vi "Status Log FGV.vi"(7 "Action":T1=enum."Show Status File", 8 "error in":errorcluster, 10 "Status":string) -> (0 "error out":errorcluster)   [LabVIEW 2016]
doc: "FGV for managing status log file"
uses:
  Status Log.ctl
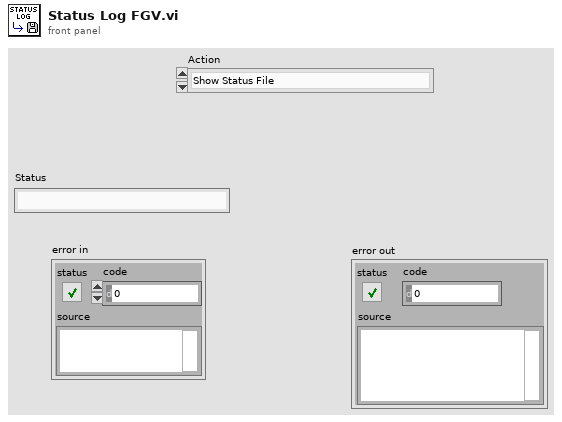
[diagram p1: front panel]
types:
  T1 = typedef "Status Log.ctl" = enum16{"Close file", "Open Status file", "Add Status", "Show Status File"}
  T2 = enum16{"open", "replace", "create", "open or create", "replace or create", "replace or create with confirmation"}
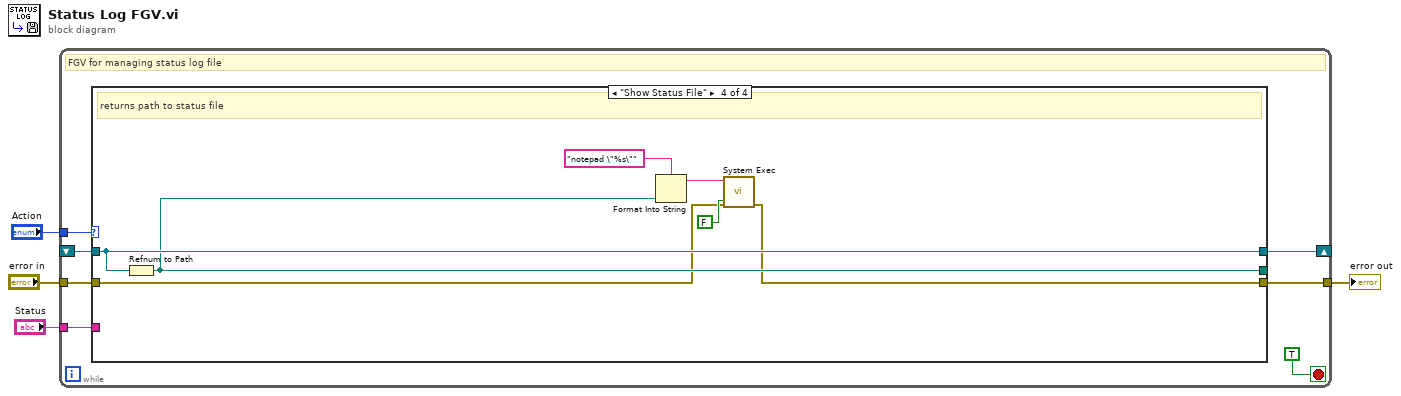
[diagram p0: block diagram]
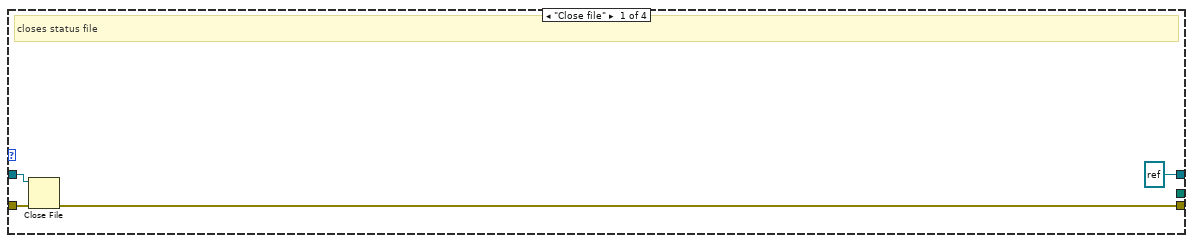
[diagram p2: hidden frame]
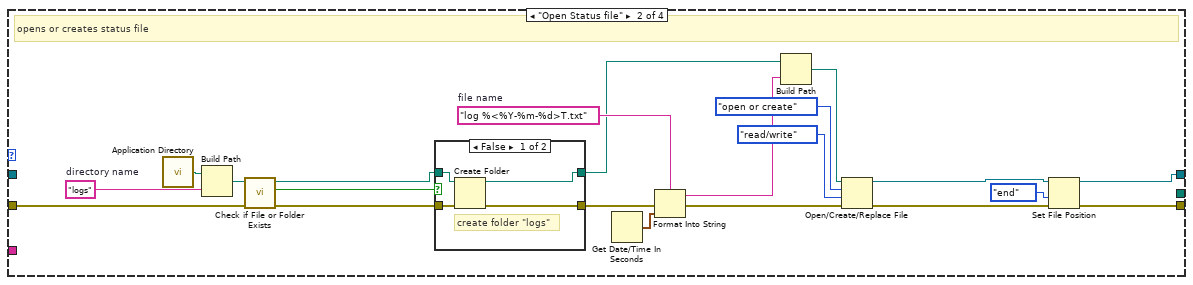
[diagram p3: hidden frame]
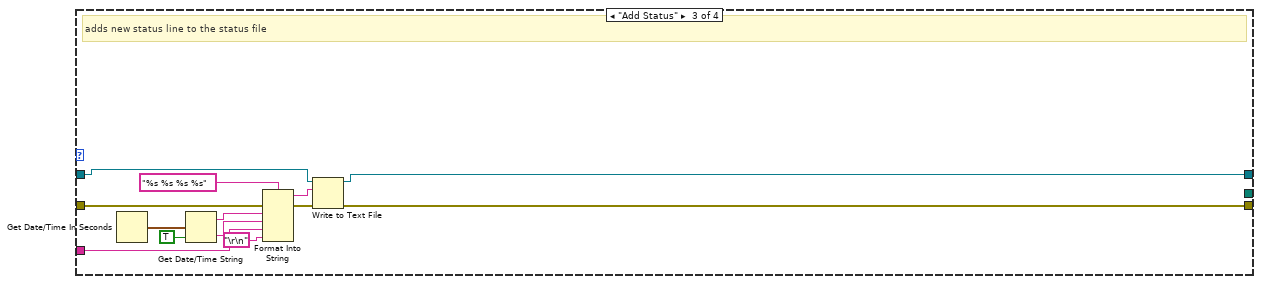
[diagram p5: hidden frame]
diagram:
  n1 = while {
    tunnel: "Action" -> [w10]
    tunnel: "Status" -> [w9]
    tunnel: [w8] -> w2
    tunnel: "error in" -> [w7]
    shift-right: [w5] -> _
    shift-left: _ -> [w6]
    stop <- TRUE stop-if-true
    # "FGV for managing status log file"
    n2 = case shown="\"Show Status File\"" w10 {
      tunnel: w9 -> [_ _ w49 _]
      tunnel: [w14 w25 w46 w56] -> w8
      tunnel: w7 -> [w15 w17 w55 w57]
      tunnel: [refnum<file> refnum ("refnum out") w24 w43 w62] -> w5
      tunnel: w6 -> [w13 _ w45 w62]
      tunnel: [_ _ _ w58] -> _
      frame "Close file" {
        # "closes status file"
        n3 = Close File(refnum=w13, error in=w15) -> (error out=w14:errorcluster)  [unwired: 1 out]
      }
      frame "Open Status file" {
        w30 = "log %<%Y-%m-%d>T.txt"  # file name
        w35 = "logs"  # directory name
        # "opens or creates status file"
        n4 = call <vilib>:"Application Directory.vi"() -> ("Application Directory"=w36:path)
        n5 = Build Path(base path=w36, name or relative path=w35) -> (appended path=w22:path)
        n6 = call <vilib>:"Check if File or Folder Exists.vi"("error in (no error)"=w17, "path"=w22) -> ("error out"=w18:errorcluster, "file or folder exists?"=w21:bool, "dup path"=w20:path)  [unwired: 7 in]
        n7 = case shown="False" w21 {
          tunnel: w20 -> [w40 w42]
          tunnel: [w39 w42] -> w19
          tunnel: w18 -> [w38 w41]
          tunnel: [w37 w41] -> w16
          frame False {
            # "create folder \"logs\""
            n8 = Create Folder(path (use dialog)=w40, error in=w38) -> (created path=w39:path, error out=w37:errorcluster)  [unwired: 1 in, 1 out]
          }
          frame True {
          }
        }
        n9 = Get Date/Time In Seconds() -> (seconds since 1Jan1904=w34:timestamp)
        n10 = Format Into String "Format Into String"(format string=w30, error in=w16, w34) -> (resulting string=w32:string, error out=w33:errorcluster)  [unwired: 1 in]
        n11 = Build Path(base path=w19, name or relative path=w32) -> (appended path=w31:path)
        n12 = Open/Create/Replace File(file path (use dialog)=w31, error in=w33, operation (0:open)=T2."open or create", access (0:read/write)=enum16{"read/write", "read-only", "write-only"}."read/write") -> (refnum out=w26:refnum<file>, error out=w27:errorcluster)  [unwired: 2 in, 1 out]
        n13 = Set File Position(refnum=w26, from (0:start)=enum16{"start", "end", "current"}."end", error in=w27) -> (refnum out=w24:refnum<file>, error out=w25:errorcluster)  [unwired: 1 in]
      }
      frame "Add Status" {
        # "adds new status line to the status file"
        n14 = Get Date/Time In Seconds() -> (seconds since 1Jan1904=w53:timestamp)
        n15 = Get Date/Time String(seconds (now)=w53, want seconds? (F)=TRUE) -> (date string=w51:string, time string=w50:string)  [unwired: 1 in]
        n16 = Format Into String(format string="%s %s %s %s", error in=w55, w51, w50, w49, "\r\n") -> (resulting string=w44:string, error out=w47:errorcluster)  [unwired: 1 in]
        n17 = Write to Text File(file (use dialog)=w45, text=w44, error in=w47) -> (refnum out=w43:refnum<file>, error out=w46:errorcluster)  [unwired: 1 in, 1 out]
      }
      frame "Show Status File" {
        # "returns path to status file"
        n18 = Refnum to Path(1:w62) -> (0:w58:path)
        n19 = Format Into String(format string="notepad \"%s\"", w58) -> (resulting string=w59:string)  [unwired: 2 in, 1 out]
        n20 = call <vilib>:"System Exec.vi"("run minimized? (F)"=FALSE, "error in (no error)"=w57, "command line"=w59) -> ("error out"=w56:errorcluster)  [unwired: 5 in, 3 out]
      }
    }
  }
  "error out" <- w2
